vi "Analyze Waveform.vi"(7 "Chart Ref":refnum<vi>) -> ()   [LabVIEW 2014]
panel:
  in  "Exit":bool
  in  "Reset Scale":bool
  in  "Log Info Button":bool
  in  "Snapshot":bool
  in  "Open Log":bool
  in  "Rescale Y":bool
  out "Cursor Delta (T2 - T1)":cluster{"X":dbl, "Y":dbl} {"Y" format="%9.3p"; "X" format="%.3g"}
  out "Cursor T2":cluster{"X":dbl, "Y":dbl} {"Y" format="%9.3p"; "X" format="%.3g"}
  out "Cursor T1":cluster{"X":dbl, "Y":dbl} {"Y" format="%9.3p"; "X" format="%.3g"}
  out "Mouse Position":cluster{"X":dbl, "Y":dbl} {"Y" format="%.3g"; "X" format="%.3g"}
  out "Analyze Signal":waveform(dbl)(graph)
  # "Analyze Waveform Signal"
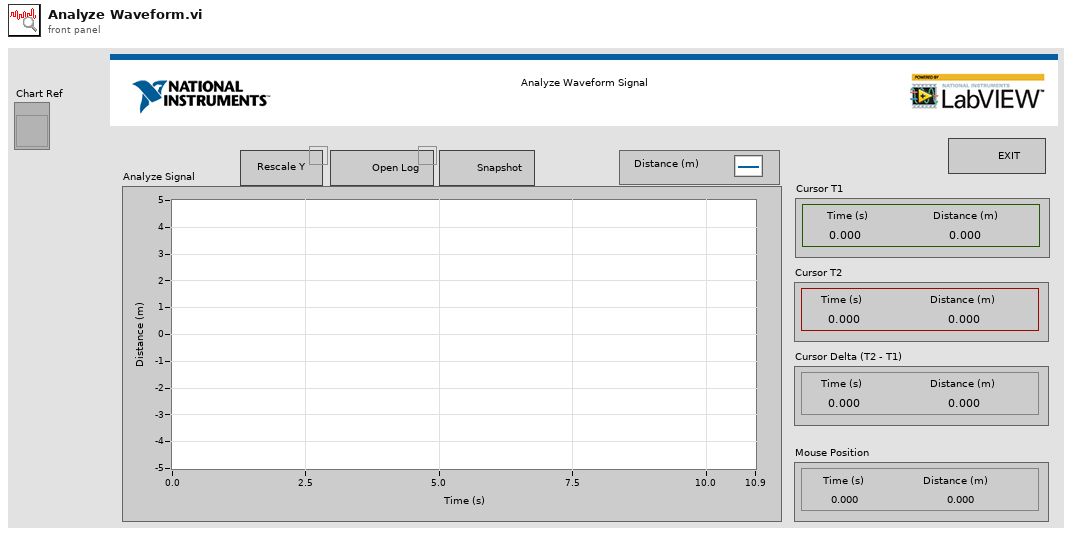
[diagram p1: front panel]
types:
  T1 = typedef "LVRangeTypeDef.ctl" = cluster{"Minimum":dbl, "Maximum":dbl, "Increment":dbl, "Minor Increment":dbl, "Start":dbl}
  T2 = typedef "LVPoint32TypeDef.ctl" = cluster{"Horizontal":i32, "Vertical":i32}
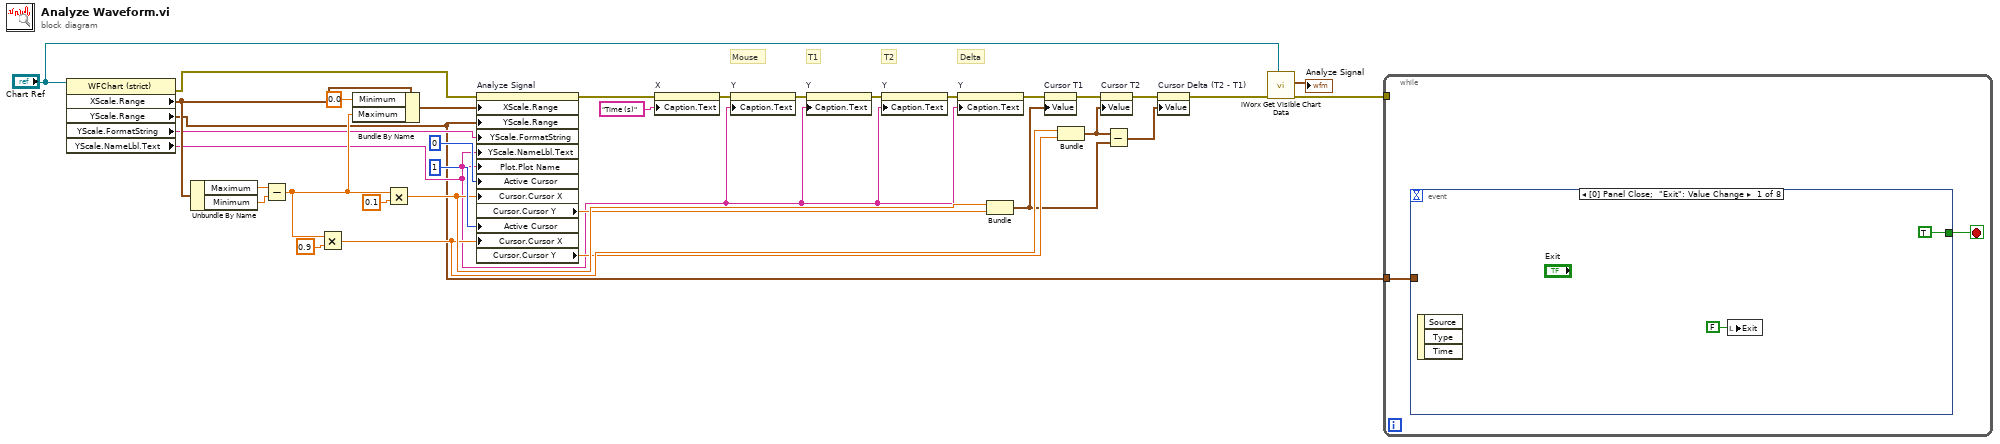
[diagram p0: block diagram]
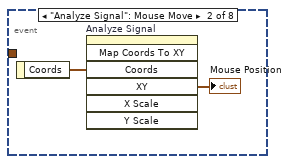
[diagram p2: hidden frame]
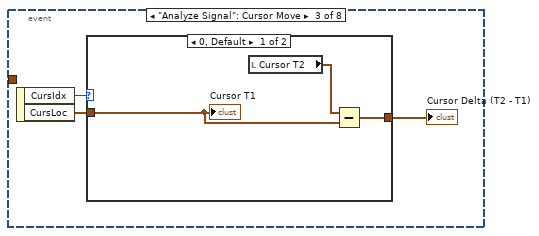
[diagram p3: hidden frame]
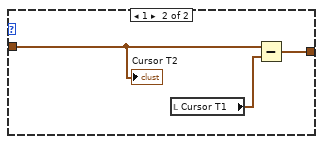
[diagram p4: hidden frame]
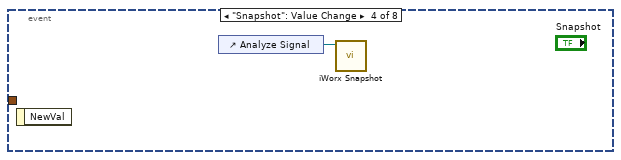
[diagram p5: hidden frame]
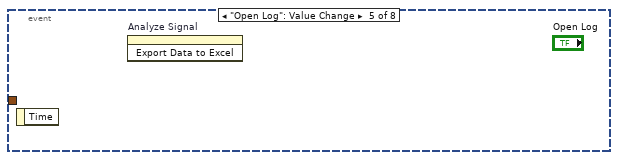
[diagram p6: hidden frame]
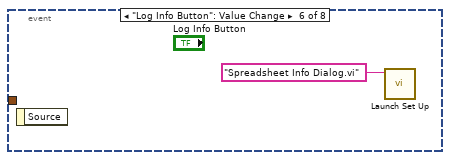
[diagram p7: hidden frame]
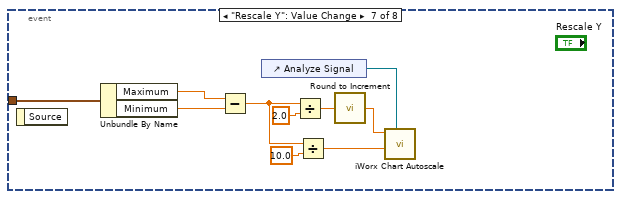
[diagram p8: hidden frame]
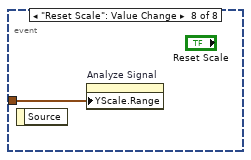
[diagram p9: hidden frame]
diagram:
  # "Delta"
  # "T2"
  # "Mouse"
  # "T1"
  n1 = property on="Property Node" class="WFChart (strict)"(reference="Chart Ref") -> (error out=w3:errorcluster, "XScale.Range"=w30:T1, "YScale.Range"=w4:T1, "YScale.FormatString"=w7:string, "YScale.NameLbl.Text"=w9:string)  [unwired: 1 in, 1 out]
  n2 = Unbundle By Name(w30) -> ("Maximum"=w32:dbl, "Minimum"=w31:dbl)
  n3 = Subtract(x=w32, y=w31) -> (x-y=w21:dbl)
  n4 = Multiply(x=w21, y=0.9) -> (x*y=w17:dbl)
  n5 = Bundle By Name(cluster=w30, "Minimum"=0.0, "Maximum"=w21) -> (w28:T1)
  n6 = Multiply(x=w21, y=0.1) -> (x*y=w20:dbl)
  n7 = property on="Analyze Signal" class="WFGraph (strict)"(error in=w3, "XScale.Range"=w28, "YScale.Range"=w4, "YScale.FormatString"=w7, "YScale.NameLbl.Text"=w9, "Plot.Plot Name"=w9, "Active Cursor"=u32 0, "Cursor.Cursor X"=w20, "Active Cursor"=u32 1, "Cursor.Cursor X"=w17) -> (error out=w6:errorcluster, "Cursor.Cursor Y"=w19:dbl, "Cursor.Cursor Y"=w16:dbl)  [unwired: 1 in, 1 out]
  n8 = property on="X" class="DigNum (strict)"(error in=w6, "Caption.Text"="Time (s)" ("Label.Text")) -> (error out=w27:errorcluster)  [unwired: 1 in, 1 out]
  n9 = property on="Y" class="DigNum (strict)"(error in=w27, "Caption.Text"=w9) -> (error out=w13:errorcluster)  [unwired: 1 in, 1 out]
  n10 = property on="Y" class="DigNum (strict)"(error in=w13, "Caption.Text"=w9) -> (error out=w12:errorcluster)  [unwired: 1 in, 1 out]
  n11 = property on="Y" class="DigNum (strict)"(error in=w12, "Caption.Text"=w9) -> (error out=w8:errorcluster)  [unwired: 1 in, 1 out]
  n12 = property on="Y" class="DigNum (strict)"(error in=w8, "Caption.Text"=w9) -> (error out=w5:errorcluster)  [unwired: 1 in, 1 out]
  n13 = Bundle(w20, "Cursor.Cursor Y"=w19) -> (w14:cluster{dbl, "Cursor.Cursor Y":dbl})  [unwired: 1 in]
  n14 = property on="Cursor T1" class="Clust (strict)"(error in=w5, "Value"=w14) -> (error out=w18:errorcluster)  [unwired: 1 in, 1 out]
  n15 = Bundle(w17, "Cursor.Cursor Y"=w16) -> (w15:cluster{dbl, "Cursor.Cursor Y":dbl})  [unwired: 1 in]
  n16 = property on="Cursor T2" class="Clust (strict)"(error in=w18, "Value"=w15) -> (error out=w11:errorcluster)  [unwired: 1 in, 1 out]
  n17 = Subtract(x=w15, y=w14) -> (x-y=w10:cluster{dbl, "Cursor.Cursor Y":dbl})
  n18 = property on="Cursor Delta (T2 - T1)" class="Clust (strict)"(error in=w11, "Value"=w10) -> (error out=w2:errorcluster)  [unwired: 1 in, 1 out]
  n19 = call "iWorx Get Visible Chart Data.vi"("Selection Chart"="Chart Ref", "Error In"=w2) -> ("Error Out"=w1:errorcluster, "Waveform out"=→"Analyze Signal":waveform(dbl))  [unwired: 7 in, 1 out]
  n20 = while {
    tunnel: w4 -> [w35]
    tunnel: w1 -> [_]
    stop <- w36 stop-if-true
    n21 = event shown="[0] Panel Close;  \"Exit\": Value Change" {
      selector: _ -> [_ _ _ _ _ _ _ _]
      dyn-events: _ -> [_ _ _ _ _ _ _ _]
      timeout: _ -> [_ _ _ _ _ _ _ _]
      tunnel: [TRUE _ _ _ _ _ _ _] -> w36
      tunnel: w35 -> [_ _ _ _ _ _ w60 w62]
      event Panel Close; "Exit": Value Change {
        n22 = event-data() -> ()  [unwired: 1 in, 3 out]
        n23 = local write "Exit"(FALSE ("Exit")) -> ()
      }
      event "Analyze Signal": Mouse Move {
        n24 = event-data() -> ("Coords"=w40:T2)  [unwired: 1 in]
        n25 = invoke on="Analyze Signal" class="WFGraph (strict)" method="Map Coords To XY"("Coords"=w40) -> ("XY"=→"Mouse Position":cluster{"X":dbl, "Y":dbl})  [unwired: 6 in, 6 out]
      }
      event "Analyze Signal": Cursor Move {
        n26 = event-data() -> ("CursIdx"=w43:i32, "CursLoc"=w42:cluster{"X":dbl, "Y":dbl})  [unwired: 1 in]
        n27 = case shown="0, Default" w43 {
          tunnel: w42 -> [w46 w48]
          tunnel: [w44 w47] -> w41
          frame 0, Default {
            n28 = local read "Cursor T2"() -> (w45:cluster{"X":dbl, "Y":dbl})
            n29 = Subtract(x=w45, y=w46) -> (x-y=w44:cluster{"X":dbl, "Y":dbl})
            "Cursor T1" <- w46
          }
          frame 1 {
            n30 = local read "Cursor T1"() -> (w49:cluster{"X":dbl, "Y":dbl})
            n31 = Subtract(x=w48, y=w49) -> (x-y=w47:cluster{"X":dbl, "Y":dbl})
            "Cursor T2" <- w48
          }
        }
        "Cursor Delta (T2 - T1)" <- w41
      }
      event "Snapshot": Value Change {
        n32 = event-data() -> ()  [unwired: 1 in, 1 out]
        n33 = control-ref of="Analyze Signal"() -> (w50:refnum<vi>)
        n34 = call "iWorx Snapshot.vi"("WaveformChart in"=w50) -> ()  [unwired: 10 in, 1 out]
      }
      event "Open Log": Value Change {
        n35 = event-data() -> ()  [unwired: 1 in, 1 out]
        n36 = invoke on="Analyze Signal" class="WFGraph (strict)" method="Export Data to Excel"() -> ()  [unwired: 3 in, 3 out]
      }
      event "Log Info Button": Value Change {
        n37 = event-data() -> ()  [unwired: 1 in, 1 out]
        n38 = call "Launch Set Up.vi"("name or relative path"="Spreadsheet Info Dialog.vi") -> ()  [unwired: 9 in, 2 out]
      }
      event "Rescale Y": Value Change {
        n39 = event-data() -> ()  [unwired: 1 in, 1 out]
        n40 = Unbundle By Name(w60) -> ("Maximum"=w58:dbl, "Minimum"=w59:dbl)
        n41 = Subtract(x=w58, y=w59) -> (x-y=w54:dbl)
        n42 = control-ref of="Analyze Signal"() -> (w61:refnum<vi>)
        n43 = Divide(x=w54, y=2.0) -> (x/y=w56:dbl)
        n44 = Divide(x=w54, y=10.0) -> (x/y=w52:dbl)
        n45 = call "Round to Increment.vi"("Input"=w56) -> ("Output"=w55:dbl)
        n46 = call "iWorx Chart Autoscale.vi"("Selection Chart"=w61, "Rounding Multiple (10)"=w52, "Min Range (1)"=w55) -> ()  [unwired: 6 in, 3 out]
      }
      event "Reset Scale": Value Change {
        n47 = event-data() -> ()  [unwired: 1 in, 1 out]
        n48 = property on="Analyze Signal" class="WFGraph (strict)"("YScale.Range"=w62) -> ()  [unwired: 2 in, 2 out]
      }
    }
  }
